vi "Modules - Machines.vi"(8 "error in":errorcluster) -> (0 "error out":errorcluster)   [LabVIEW 2019]
uses:
  Controls/Machine - Device Type.ctl
  Controls/Machine-state.ctl
  <vilib>/Utility/miscctls.llb/LVRowAndColumnTypeDef.ctl
  Controls/eFGV States.ctl
  Controls/UDP - Command.ctl
  Controls/FGV States.ctl
  Controls/Communication - Write Data.ctl
  Controls/Global - Data UDP.vi
  Controls/Global - IP Address.vi
  Controls/Global - Handle V1.vi
  Controls/Global - Device.vi
  Controls/Global - Comport.vi
  Controls/Global - Channel.vi
  Controls/Global - Unit.vi
  Controls/Global - Device Type.vi
  Controls/Global - Handle.vi
  Controls/Global - Rendezvous.vi
panel:
  out "Enum 2":T1
  out "Numeric":i32
  out "Status out":string[](array[string])
  out "Enum":T1
  out "Loop":i32
  out "Success":bool
  out "Which Button?":T2(ring)=enum."Center Button"
  in  "Settings":bool
  out "Device Type":string[](array[string])
  out "Device IP":string[](array[string])
  out "Label Ch2":string caption="Cell Pressure Transducer"
  out "Label Ch1":string caption="Cell Pressure Transducer"
  out "Channel 2":sgl format="%.2f"
  out "Channel 1":sgl caption="Kpa" format="%.3f"
  out "Label Ch4":string caption="Cell Pressure Transducer"
  out "Label Ch3":string caption="Cell Pressure Transducer"
  out "Channel 3":sgl format="%.2f"
  out "Channel 4":sgl caption="Kpa" format="%.2f"
  out "error out 2":errorcluster
  in  "Remove":bool
  in  "Add":bool
  in  "Table":i32(listbox)
  out "Main Tab":enum32{"Blank", "Edit"}(tab)
  in  "Machine Setting":bool
  out "Array":cluster{"Label":string, "Data":string}[](array[cluster])
  in  "Device Type":T3 items=["Unitron", "Flowtron", "Datalogger"]
  in  "Port":string
  in  "Device IP Address/SN":string
  in  "Device Name":string
  in  "Save Edit":bool
  in  "Refresh Button":bool
  in  "Reconnect":bool
  # "*Double-Click to Edit"
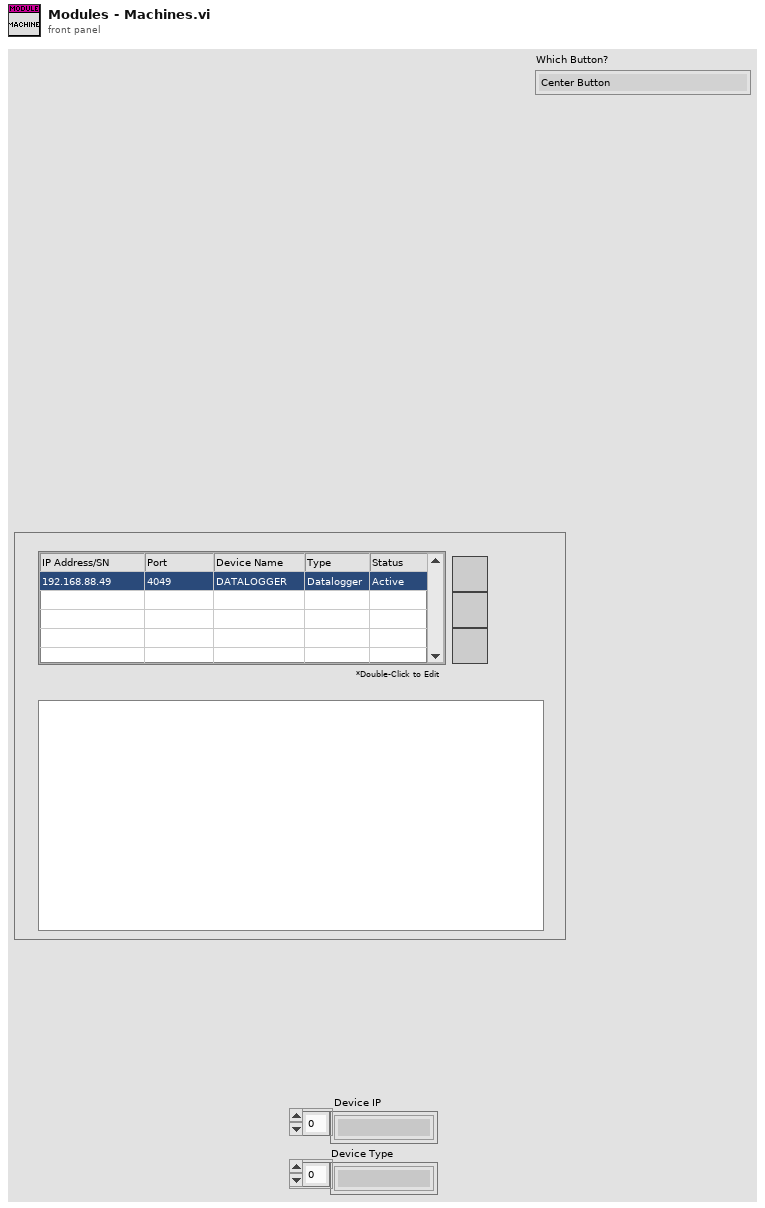
[diagram p1: front panel]
types:
  T1 = typedef "Machine-state.ctl" = enum16{"Init", "Read DB", "Read", "Idle", "Update", "Reset", "Close", "Exit"}
  T2 = enum16{"Left Button", "Center Button", "Right Button", "Window Close"}
  T3 = typedef "Machine - Device Type.ctl" = u16
  T4 = cluster{"Table":string[][], "no id":string, "doubleclick?":bool, "Timeout":i32, "Edit row":i32, "reset":i32}
  T5 = typedef "FGV States.ctl" = enum16{"Read", "Write"}
  T6 = enum32{"Invalid", "Standard", "Closed", "Hidden", "Minimized", "Maximized"}
  T7 = cluster{"Name":string[], "Unit":string[], "Decimal Point":u8[], "Ch Log":u8[], "H Alarm":u8[], "L Alarm":u8[], "H Limit":sgl[], "L Limit":sgl[], "Filter":u8[], "Gain":u8[], "Calib Type":u32[]}
  T8 = typedef "UDP - Command.ctl" = enum16{"Stop", "Jog Up", "Jog Down", "Ramp Up", "Ramp Down", "PID Target", "PID Ramp", "Disp Run", "Read Ch Data", "Zero Channel", "Zero Disp", "Read Sensor", "Write Sensor", "Read ADC", "Write ADC", "Read PID", "Write PID", "Read Test", "Write Test", "Read System", "Write System", "Read Datalog", "Read Datalog Sensor"}
  T9 = typedef "Communication - Write Data.ctl" = cluster{"Test":cluster{"Target Load":sgl, "Target Disp":sgl, "Rate":sgl, "Speed":sgl}, "Sensor":cluster{"Name":string[], "Unit":string[], "Decimal Point":u8[], "Ch Log":u8[], "H Alarm":u8[], "L Alarm":u8[], "H Limit":sgl[], "L Limit":sgl[], "Filter":u8[], "Gain":u8[], "Calib Type":u32[]}, "PID":cluster{"SP":sgl, "PV":sgl, "kP":sgl, "kI":sgl, "kD":sgl, "FF":sgl, "Err Band":sgl, "Max":i32, "Min":i32, "Ts":u32, "Out":i32, "Mode":u8}, "ADC":cluster{"Active Ch":u8[], "Filter Type":u8, "Post Filter":u8[], "Gain":u8[], "FS":u16, "IntOC":u8, "IntFC":u8, "SysOC":u8, "Cofficient":dbl[], "K":dbl[], "Max":i32}, "System":cluster{"Out Type":u8, "Inverse":u8, "Monitor":u8, "Reserve":u8, "ACC Time":u32, "Pulse Rev":u32, "Stroke":u32, "Auto Off":u32, "Gear Ratio":sgl, "Pitch":sgl, "Max Speed":u32, "Jog Speed":u32, "Disp Coff":sgl, "Max Load":u32}, "Index":enum16{"Ch1", "Ch2", "Ch3", "Ch4", "Ch5", "Ch6", "Ch7", "Ch8", "Ch9", "Ch10", "Ch11", "Ch12", "Ch13", "Ch14", "Ch15", "Ch16"}, "Datalog":enum16{"Ch1-Ch16", "Ch17-Ch32", "Ch32-Ch48", "Ch49-Ch64", "Empty"}}
  T10 = typedef "eFGV States.ctl" = enum16{"Init", "Read", "Write", "Exit"}
  T11 = typedef "Rendezvous RefNum" = refnum<k1>
  T12 = typedef "UDP - Event.ctl" = u16
  T13 = typedef "UDP - Status.ctl" = u16
  T14 = cluster{"Channels":cluster{"Ch1":sgl, "Ch2":sgl, "Ch3":sgl, "Ch4":sgl, "Ch5":sgl, "Ch6":sgl, "Ch7":sgl, "Ch8":sgl, "Ch9":sgl, "Ch10":sgl, "Ch11":sgl, "Ch12":sgl, "Ch13":sgl, "Ch14":sgl, "Ch15":sgl, "Ch16":sgl}, "Event":T12, "Status":T13, "IP":string}[]
  T15 = cluster{"Channels":cluster{"Ch1":sgl, "Ch2":sgl, "Ch3":sgl, "Ch4":sgl, "Ch5":sgl, "Ch6":sgl, "Ch7":sgl, "Ch8":sgl, "Ch9":sgl, "Ch10":sgl, "Ch11":sgl, "Ch12":sgl, "Ch13":sgl, "Ch14":sgl, "Ch15":sgl, "Ch16":sgl}, "Event":T12, "Status":T13, "IP":string}
  T16 = cluster{"Name":string[], "Unit":string[], "Decimal Point":u8[], "Ch Log":u8[], "H Alarm":u8[], "L Alarm":u8[], "H Limit":sgl[], "L Limit":sgl[], "Filter":u8[], "Gain":u8[], "Calib Type":u32[]}[]
  T17 = cluster{"Ch1":sgl, "Ch2":sgl, "Ch3":sgl, "Ch4":sgl, "Ch5":sgl, "Ch6":sgl, "Ch7":sgl, "Ch8":sgl, "Ch9":sgl, "Ch10":sgl, "Ch11":sgl, "Ch12":sgl, "Ch13":sgl, "Ch14":sgl, "Ch15":sgl, "Ch16":sgl}
  T18 = cluster{"Ch1 Unit":string, "Ch2 Unit":string, "Ch1 Decimal":u8, "Ch2 Decimal":u8, "Ch1 Cal Type":u8, "Ch2 Cal Type":u8}
  T19 = cluster{"IP Address":string, "port":string, "UDP ref":refnum<k16>}[]
  T20 = cluster{"IP Address":string, "port":string, "UDP ref":refnum<k16>}
  T21 = cluster{"Test":cluster{"Target Load":sgl, "Target Disp":sgl, "Rate":sgl, "Speed":sgl}, "Sensor":cluster{"Name":string[], "Unit":string[], "Decimal Point":u8[], "Ch Log":u8[], "H Alarm":u8[], "L Alarm":u8[], "H Limit":sgl[], "L Limit":sgl[], "Filter":u8[], "Gain":u8[], "Calib Type":u32[]}, "PID":cluster{"SP":sgl, "PV":sgl, "kP":sgl, "kI":sgl, "kD":sgl, "FF":sgl, "Err Band":sgl, "Max":i32, "Min":i32, "Ts":u32, "Out":i32, "Mode":u8}, "ADC":cluster{"Active Ch":u8[], "Filter Type":u8, "Post Filter":u8[], "Gain":u8[], "FS":u16, "IntOC":u8, "IntFC":u8, "SysOC":u8, "Cofficient":dbl[], "K":dbl[], "Max":i32}, "Status":T13, "Event":T12, "System":cluster{"Out Type":u8, "Inverse":u8, "Monitor":u8, "Reserve":u8, "ACC Time":u32, "Pulse Rev":u32, "Stroke":u32, "Auto Off":u32, "Gear Ratio":sgl, "Pitch":sgl, "Max Speed":u32, "Jog Speed":u32, "Disp Coff":sgl, "Max Load":u32}, "Channels":cluster{"Ch1":sgl, "Ch2":sgl, "Ch3":sgl, "Ch4":sgl, "Ch5":sgl, "Ch6":sgl, "Ch7":sgl, "Ch8":sgl, "Ch9":sgl, "Ch10":sgl, "Ch11":sgl, "Ch12":sgl, "Ch13":sgl, "Ch14":sgl, "Ch15":sgl, "Ch16":sgl}}
  T22 = typedef "LVRowAndColumnTypeDef.ctl" = cluster{"Row":i32, "Column":i32}
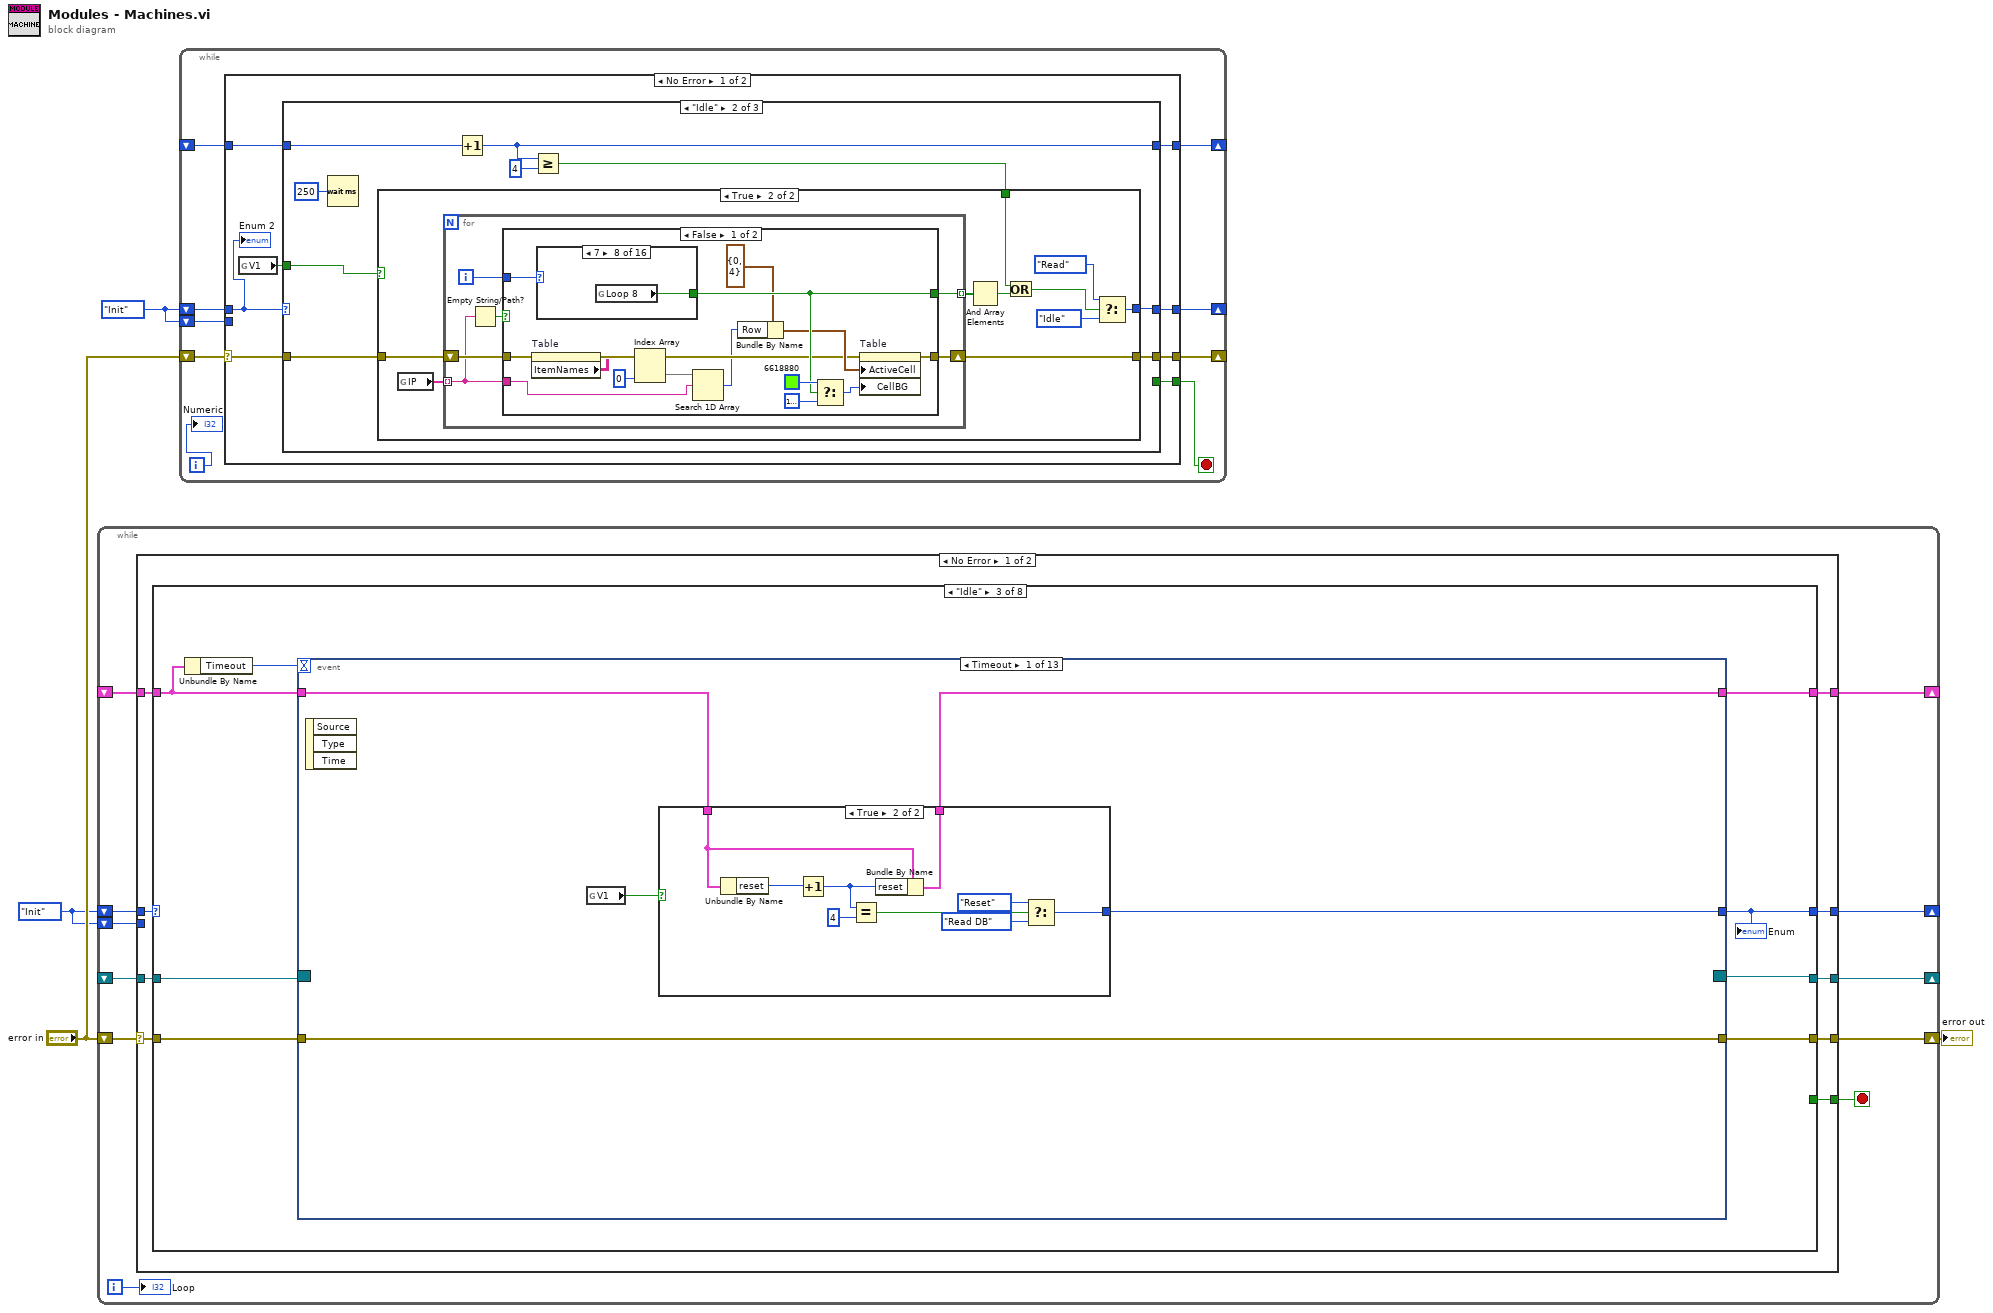
[diagram p0: block diagram]
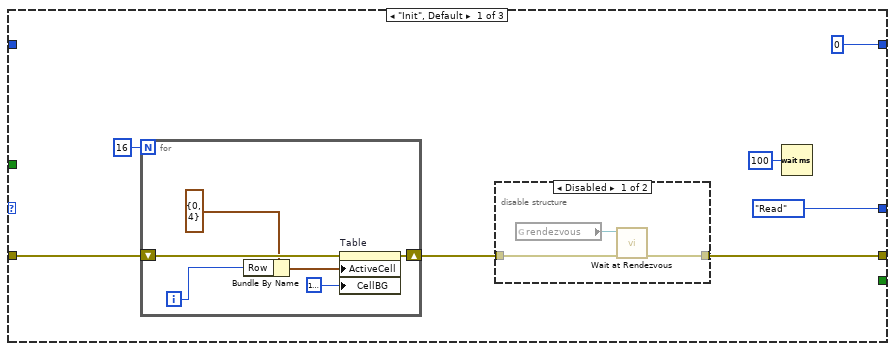
[diagram p2: hidden frame]
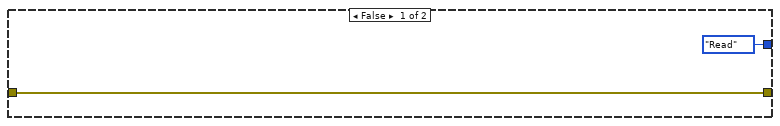
[diagram p4: hidden frame]
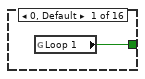
[diagram p5: hidden frame]
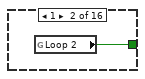
[diagram p6: hidden frame]
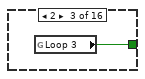
[diagram p7: hidden frame]
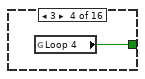
[diagram p8: hidden frame]
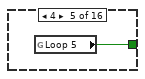
[diagram p9: hidden frame]
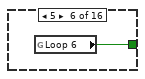
[diagram p10: hidden frame]
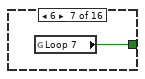
[diagram p11: hidden frame]
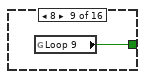
[diagram p12: hidden frame]
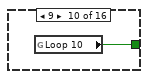
[diagram p13: hidden frame]
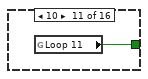
[diagram p14: hidden frame]
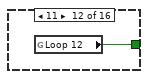
[diagram p15: hidden frame]
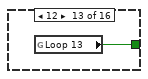
[diagram p16: hidden frame]
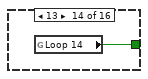
[diagram p17: hidden frame]
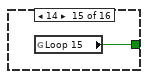
[diagram p18: hidden frame]
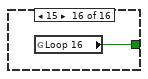
[diagram p19: hidden frame]
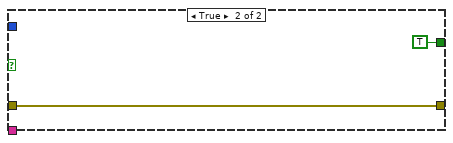
[diagram p20: hidden frame]
diagram:
  w1 = Machine-state."Init"
  w2 = Machine-state."Init"
  n1 = while {
    shift-right: [w14] -> w4
    shift-left: "error in" -> [w15]
    shift-right: [w12] -> _
    shift-left: w2 -> [w13]
    shift-right: [w10] -> _
    shift-left: _ -> [w9]
    shift-right: [w8] -> _
    shift-left: _ -> [w7]
    shift-left: w2 -> [w5]
    i -> [w6]
    stop <- w11 stop-if-true
    n2 = case shown="No Error" w15 {
      selector: w15 -> [w20 w611]
      tunnel: [w21 w612] -> w14
      tunnel: w13 -> [w24 _]
      tunnel: [w23 Machine-state."Idle"] -> w12
      tunnel: [w22 _] -> w11
      tunnel: [w19 w617] -> w10
      tunnel: w9 -> [w18 w617]
      tunnel: [w17 w614] -> w8
      tunnel: w7 -> [w16 w614]
      tunnel: w5 -> [_ w603]
      frame No Error {
        n3 = case shown="\"Idle\"" w24 {
          tunnel: [Machine-state."Read DB" Machine-state."Read" w127 Machine-state."Idle" Machine-state."Read DB" Machine-state."Idle" Machine-state."Idle" Machine-state."Exit"] -> w23
          tunnel: [_ _ _ _ _ _ FALSE TRUE] -> w22
          tunnel: [w39 w57 w129 w397 w477 w484 w588 w598] -> w21
          tunnel: w20 -> [w26 w75 w128 w401 w461 w483 w592 w597]
          tunnel: [T4 {"Table"=[], "no id"="", "doubleclick?"=FALSE, "Timeout"=1000, "Edit row"=-1, "reset"=0} w79 w126 w403 w472 w487 w591 w602] -> w19
          tunnel: w18 -> [_ w78 w123 w402 w472 w487 w591 w602]
          tunnel: [w36 w80 w124 w411 w482 w485 w589 w601] -> w17
          tunnel: w16 -> [_ w80 w125 w411 w482 w485 w589 w601]
          frame "Init", Default {
            w30 = eFGV_States."Read" ("Action")
            n4 = global read "Global - Data UDP.vi" "V1"() -> (w25:bool)
            n5 = property on="Reconnect" class="Bool"(error in=w26, "Visible"=w25) -> (error out=w27:errorcluster)  [unwired: 1 in, 1 out]
            n6 = Not(x=w25) -> (.not. x?=w28:bool)
            n7 = property on="Device Type" class="Ring (strict)"(error in=w27, "Visible"=w28) -> (error out=w29:errorcluster)  [unwired: 1 in, 1 out]
            n8 = disable-structure shown="Enabled" {
              disable-tunnel: w29 -> [w45 w47]
              disable-tunnel: [w44 w47] -> w33
              frame Disabled {
                n9 = global read "Global - Rendezvous.vi" "rendezvous"() -> (w46:T11)
                n10 = call <vilib>:"Wait at Rendezvous.vi"("error in (no error)"=w45, "rendezvous"=w46) -> ("error out"=w44:errorcluster)  [unwired: 3 in, 2 out]
              }
              frame Enabled {
              }
            }
            n11 = local write "Device Name"("" ("New machine name")) -> ()
            n12 = call "Main - Minimized (eFGV).vi"("Action"=w30, "error in"=w33) -> ("error out"=w32:errorcluster, "Minimized ref"=w31:refnum<user-event>)  [unwired: 7 in, 1 out]
            n13 = call "Communication - Trigger Read IP Address(FGV).vi"("Action"=w30, "error in"=w32) -> ("error out"=w35:errorcluster, "Trigger ref"=w34:refnum<user-event>)  [unwired: 7 in, 1 out]
            n14 = call "General - Exit eFGV.vi"("eFGV States"=w30, "error in (no error)"=w35) -> ("error out"=w40:errorcluster, "Exit"=w38:refnum<user-event>)  [unwired: 7 in, 1 out]
            n15 = register-events(error in=w40, w38, w34, w31) -> (reference out=w36:refnum<event-registration>, error out=w39:errorcluster)  [unwired: 1 in]
            "Main Tab" <- enum32{"Blank", "Edit"}."Blank" ("Main Tab")
          }
          frame "Read DB" {
            n16 = global read "Global - IP Address.vi" "IP"() -> (w48:string[])
            n17 = global read "Global - Data UDP.vi" "V1"() -> (w50:bool)
            n18 = call "Machine - Config File.vi"("Action"=enum16{"Write", "Read", "Read All", "Remove"}."Read All", "V1"=w50, "error in (no error)"=w75) -> ("error out"=w71:errorcluster, "Value Out"=w76:cluster{"IP/SN":string, "Key Value":string[]}[])  [unwired: 7 in]
            n19 = for {
              tunnel: [w113] -> w74 mode=indexing
              tunnel: w76 -> [w109] mode=indexing
              tunnel: [w102] -> w72 mode=indexing
              shift-right: [w107] -> w70
              shift-left: w71 -> [w108]
              tunnel: w48 -> [w94]
              n20 = Unbundle(w109) -> ("IP/SN"=w102:string, "Key Value"=w112:string[])
              n21 = Index Array(array=w112) -> (element #1=w101:string, element #2=w100:string, element #3=w93:string, element #4=w97:string)  [unwired: 4 in]
              n22 = Search 1D Array(1D array=w94, element=w102) -> (index of element=w96:i32)  [unwired: 1 in]
              n23 = Less Than 0?(x=w96) -> (x < 0?=w99:bool)
              n24 = Select(t="1" ("y"), s=w99, f="0") -> (s? t:f=w92:string)
              n25 = Select(t="Disable" ("y"), s=w99, f="Active" ("y")) -> (s? t:f=w98:string)
              n26 = Equal?(x=w92, y=w93) -> (x = y?=w91:bool)
              n27 = global read "Global - Data UDP.vi" "V1"() -> (w95:bool)
              n28 = Build Array(w92) -> (w103:string[])
              n29 = case shown="False" w91 {
                tunnel: w108 -> [w119 w121]
                tunnel: [w118 w121] -> w107
                tunnel: string[] ["Status"] ("Key Name") -> [w117 _]
                tunnel: w103 -> [w116 _]
                tunnel: w102 -> [w115 _]
                tunnel: w95 -> [w114 _]
                frame False {
                  n30 = call "Machine - Config File.vi"("Action"=enum16{"Write", "Read", "Read All", "Remove"}."Write", "V1"=w114, "error in (no error)"=w119, "Value"=w116, "Key Name"=w117, "IP/SN"=w115) -> ("error out"=w118:errorcluster)  [unwired: 4 in, 1 out]
                }
                frame True {
                }
              }
              n31 = Build Array(w101, w100, w97, w98) -> (w113:string[])
            }
            n32 = Empty Array?(array=w74) -> ()  [unwired: 1 out]
            n33 = case shown="False" FALSE {
              tunnel: [w85 w89] -> w68
              tunnel: w74 -> [w84 _]
              tunnel: [w83 w90] -> w73
              tunnel: w70 -> [w83 w90]
              tunnel: w72 -> [w82 _]
              frame False {
                n34 = Transpose 2D Array(2D array=w84) -> (transposed array=w86:string[][])
                n35 = Build Array (concatenate)(w82, w86) -> (w87:string[][])
                n36 = Transpose 2D Array(2D array=w87) -> (transposed array=w85:string[][])
              }
              frame True {
                n37 = global read "Global - IP Address.vi" "IP"() -> (w88:string[])
                n38 = Build Array(w88) -> (w89:string[][])
              }
            }
            n39 = property on="Table" class="MCListbox (strict)"(error in=w73, "ItemNames"=w68) -> (error out=w65:errorcluster)  [unwired: 1 in, 1 out]
            n40 = Bundle By Name(cluster=w78, "Table"=w68) -> (w79:T4)
            n41 = Index Array(array=w68, index (col) #1=3 ("disabled index (col)"), index (col) #2=0 ("disabled index (col)"), index (col) #3=2 ("disabled index (col)"), index (col) #4=4 ("index (col)")) -> (element #1=→"Device Type":string[], element #2=w53:string[], element #3=w62:string[], element #4=w63:string[])  [unwired: 4 in]
            "Device IP" <- w53
            n42 = call "Main - Machine Connectivity (FGV).vi"("Action"=FGV_States."Write", "error In"=w65, "Status"=w63, "Device Name"=w62) -> ("error out"=w58:errorcluster, "Status out"=→"Status out":string[])  [unwired: 5 in, 1 out]
            n43 = call "Communication - Heartbeat (FGV).vi"("Action"=FGV_States."Read", "error in (no error)"=w58) -> ("error out"=w59:errorcluster, "Previous Out"=w55:string[], "Timestamp Out"=w56:string[])  [unwired: 6 in, 1 out]
            n44 = call "Communication - Heartbeat (FGV).vi"("Action"=FGV_States."Write", "error in (no error)"=w59, "Previous"=w55, "Timestamp"=w56, "IP"=w53) -> ("error out"=w57:errorcluster)  [unwired: 3 in, 3 out]
          }
          frame "Idle" {
            n45 = Unbundle By Name(w123) -> ("Timeout"=w122:i32)
            n46 = event shown="[0] Timeout" {
              selector: w125 -> [_ _ _ _ _ _ _ _ _ _ _ _ _]
              dyn-events: [_ _ _ _ _ _ _ _ _ _ _ _ _] -> w124
              timeout: w122 -> [_ _ _ _ _ _ _ _ _ _ _ _ _]
              tunnel: [w134 w148 w149 w159 w169 w182 w211 w223 w241 w252 w326 w360 w388] -> w129
              tunnel: w128 -> [w134 w148 w150 w159 w168 w183 w211 w224 w242 w251 w340 w359 w388]
              tunnel: [w131 Machine-state."Close" Machine-state."Idle" Machine-state."Read DB" w170 Machine-state."Idle" Machine-state."Reset" w225 Machine-state."Read DB" Machine-state."Idle" Machine-state."Idle" Machine-state."Idle" Machine-state."Exit"] -> w127
              tunnel: w123 -> [w132 w147 w155 w158 w166 w184 w208 w222 w240 w265 w343 w362 w387]
              tunnel: [w133 w147 w155 w158 w166 w185 w209 w222 w240 w265 w343 w362 w387] -> w126
              event Timeout {
                n47 = event-data() -> ()  [unwired: 1 in, 3 out]
                n48 = global read "Global - Data UDP.vi" "V1"() -> (w130:bool)
                n49 = case shown="True" w130 {
                  tunnel: [w135 w143] -> w133
                  tunnel: w132 -> [w135 w142]
                  tunnel: [Machine-state."Read DB" w138] -> w131
                  frame False {
                  }
                  frame True {
                    n50 = Unbundle By Name(w142) -> ("reset"=w145:i32)
                    n51 = Increment(x=w145) -> (x+1=w141:i32)
                    n52 = Equal?(x=w141, y=4) -> (x = y?=w140:bool)
                    n53 = Bundle By Name(cluster=w142, "reset"=w141) -> (w143:T4)
                    n54 = Select(t=Machine-state."Reset", s=w140, f=Machine-state."Read DB") -> (s? t:f=w138:T1)
                  }
                }
              }
              event Panel Close {
                n55 = event-data() -> ()  [unwired: 1 in, 4 out]
              }
              event User Event {
                n56 = event-data() -> ()  [unwired: 1 in, 5 out]
                n57 = control-ref of="This VI"() -> (w153:refnum<vi>)
                n58 = property class="VI"(reference=w153, error in=w150, "FP.State"=T6."Minimized" ("Front Panel Window:State")) -> (error out=w151:errorcluster)  [unwired: 1 out]
                n59 = call <vilib>:"Clear Errors.vi"("error in (no error)"=w151) -> ("error out"=w149:errorcluster)  [unwired: 5 in, 1 out]
              }
              event User Event {
                n60 = event-data() -> ()  [unwired: 1 in, 5 out]
                n61 = Wait (ms)(milliseconds to wait=u32 3000) -> ()  [unwired: 1 out]
              }
              event "Save Edit": Value Change {
                n62 = event-data() -> ()  [unwired: 1 in, 1 out]
                n63 = Unbundle By Name(w166) -> ("Table"=w165:string[][])
                n64 = Index Array(array=w165, index (col)=1 ("disabled index (col)")) -> (element=w162:string[])  [unwired: 1 in]
                n65 = To Upper Case(1:"Device Name") -> (0:w161:string)
                n66 = Search 1D Array(1D array=w162, element=w161) -> (index of element=w160:i32)  [unwired: 1 in]
                n67 = case shown="-1" w160 {
                  tunnel: [w174 w181] -> w169
                  tunnel: w168 -> [w174 w181]
                  tunnel: [FALSE ("T button?") w177] -> w167
                  frame 0, Default {
                    n68 = One Button Dialog(message="This machine name already exist. Please give new name", button name ("OK")="Ok") -> ()  [unwired: 1 out]
                  }
                  frame -1 {
                    n69 = Two Button Dialog(message="Are you sure?", 1:"No" ("F button name (\"Cancel\")"), 2:"Yes" ("T button name (\"OK\")")) -> (T button?=w177:bool)
                  }
                }
                n70 = Select(t=Machine-state."Update", s=w167, f=Machine-state."Idle") -> (s? t:f=w170:T1)
              }
              event "Table": Mouse Down {
                n71 = event-data() -> ("Mods.Double Click"=w187:bool)  [unwired: 1 in]
                n72 = case shown="True" w187 {
                  tunnel: w184 -> [w189 w192]
                  tunnel: [w189 w193] -> w185
                  tunnel: w183 -> [w188 w200]
                  tunnel: [w188 w200] -> w182
                  frame False {
                  }
                  frame True {
                    n73 = Unbundle By Name(w192) -> ("Table"=w203:string[][])
                    n74 = Index Array(array=w203, index (row) #1="Table", index (col) #1=0 ("disabled index (col)"), index (row) #2="Table", index (col) #2=1 ("disabled index (col)"), index (row) #3="Table", index (col) #3=2 ("disabled index (col)"), index (row) #4="Table", index (col) #4=3 ("disabled index (col)")) -> (element #1=w194:string, element #2=w190:string, element #3=w199:string, element #4=w196:string)
                    n75 = case shown="\"Datalogger\"" w196 {
                      tunnel: [w205 w206 w207] -> w195
                      frame "Unitron", Default {
                        w205 = T3 0 items=["Unitron", "Flowtron", "Datalogger"] ("Device Type")
                      }
                      frame "Flowtron" {
                        w206 = T3 1 items=["Unitron", "Flowtron", "Datalogger"] ("Device Type")
                      }
                      frame "Datalogger" {
                        w207 = T3 2 items=["Unitron", "Flowtron", "Datalogger"] ("Device Type")
                      }
                    }
                    n76 = local write "Device IP Address/SN"(w194) -> ()
                    n77 = local write "Device Name"(w199) -> ()
                    n78 = local write "Port"(w190) -> ()
                    n79 = Bundle By Name(cluster=w192, "Edit row"="Table") -> (w193:T4)
                    n80 = local write "Device Type"(w195) -> ()
                    n81 = local write "Main Tab"(enum32{"Blank", "Edit"}."Edit" ("Main Tab")) -> ()
                  }
                }
              }
              event "Refresh Button": Value Change {
                n82 = event-data() -> ()  [unwired: 1 in, 6 out]
                n83 = Bundle By Name(cluster=w208, "Timeout"=1000) -> (w209:T4)
              }
              event "Add": Value Change {
                n84 = event-data() -> ()  [unwired: 1 in, 6 out]
                n85 = Unbundle By Name(w222) -> ("Table"=w217:string[][])
                n86 = Array Size(array=w217) -> (size(s)=w221:i32[])
                n87 = Index Array(array=w221) -> (element=w220:i32)  [unwired: 1 in]
                n88 = Index Array(array=w217, index (col) #1=1 ("disabled index (col)"), index (col) #2=0 ("index (col)")) -> (element #1=w213:string[], element #2=w214:string[])  [unwired: 2 in]
                n89 = Greater Or Equal?(x=w220, y=16) -> (x >= y?=w218:bool)
                n90 = case shown="False" w218 {
                  tunnel: [Machine-state."Read DB" Machine-state."Idle"] -> w225
                  tunnel: w224 -> [w229 w232]
                  tunnel: [w228 w232] -> w223
                  tunnel: w214 -> [w227 _]
                  tunnel: w213 -> [w226 _]
                  frame False {
                    n91 = call "Machine - Add Device (SubVI).vi"("error in"=w229, "IP Address/SN"=w227, "Port"=w226) -> ("error out"=w228:errorcluster)  [unwired: 8 in]
                  }
                  frame True {
                    n92 = One Button Dialog(message="Maximum devices already reached") -> ()  [unwired: 1 in, 1 out]
                  }
                }
              }
              event "Remove": Value Change {
                n93 = event-data() -> ()  [unwired: 1 in, 6 out]
                n94 = local read "Table"() -> (w237:i32)
                n95 = Unbundle By Name(w240) -> ("Table"=w239:string[][])
                n96 = Two Button Dialog(message="Are your sure?") -> (T button?=w235:bool)  [unwired: 2 in]
                n97 = Index Array(array=w239, index (row)=w237, index (col)=0 ("disabled index (col)")) -> (element=w236:string)
                n98 = case shown="True" w235 {
                  tunnel: w242 -> [w244 w248]
                  tunnel: [w244 w247] -> w241
                  tunnel: w236 -> [_ w246]
                  frame False {
                  }
                  frame True {
                    n99 = global read "Global - Data UDP.vi" "V1"() -> (w245:bool)
                    n100 = call "Machine - Config File.vi"("Action"=enum16{"Write", "Read", "Read All", "Remove"}."Remove", "V1"=w245, "error in (no error)"=w248, "IP/SN"=w246) -> ("error out"=w247:errorcluster)  [unwired: 6 in, 1 out]
                  }
                }
              }
              event "Settings": Value Change {
                n101 = event-data() -> ()  [unwired: 1 in, 6 out]
                n102 = global read "Global - Data UDP.vi" "V1"() -> (w262:bool)
                n103 = Select(t="USB" ("message"), s=w262, f="LAN" ("message")) -> (s? t:f=w259:string)
                n104 = Format Into String(format string="Currently the system run \"%s\" communication protocol.\nSelect the Communication protocol you want to use." ("message"), initial string="", w259) -> (resulting string=w257:string)  [unwired: 1 in, 1 out]
                n105 = call <vilib>:"Three Button Dialog.vi"("Justify Message (Left)"=enum16{"Left", "Center", "Right"}."Center", "Window Title (\"\")"="Communication Protocol" ("Window Title (\"\")"), "Center Button Text (\"No\")"="LAN" ("Center Button Text (\"No\")"), "Left Button Text (\"Yes\")"="USB" ("Left Button Text (\"Yes\")"), "message"=w257) -> ("Which Button?"=w250:T2)  [unwired: 6 in]
                "Which Button?" <- w250
                n106 = case shown="\"Right Button\"" w250 {
                  tunnel: [w272 w280 w283 w304] -> w252
                  tunnel: w251 -> [w271 w279 w283 w304]
                  frame "Center Button", Default {
                    n107 = call "Machine - Config File.vi"("Setting"=TRUE, "Action"=enum16{"Write", "Read", "Read All", "Remove"}."Write", "error in (no error)"=w271, "Value"=string[] ["V2"], "Key Name"=string[] ["Controller"], "IP/SN"="Setting") -> ("error out"=w272:errorcluster)  [unwired: 4 in, 1 out]
                    n108 = One Button Dialog(message="Restart the sytem to enable the changes.") -> ()  [unwired: 1 in, 1 out]
                  }
                  frame "Left Button" {
                    n109 = call "Machine - Config File.vi"("Setting"=TRUE, "Action"=enum16{"Write", "Read", "Read All", "Remove"}."Write", "error in (no error)"=w279, "Value"=string[] ["V1"], "Key Name"=string[] ["Controller"], "IP/SN"="Setting") -> ("error out"=w280:errorcluster)  [unwired: 4 in, 1 out]
                    n110 = One Button Dialog(message="Restart the sytem to enable the changes.") -> ()  [unwired: 1 in, 1 out]
                  }
                  frame "Right Button" {
                    n111 = global read "Global - IP Address.vi" "IP"() -> (w282:string[])
                    n112 = for {
                      tunnel: w282 -> [w284] mode=indexing
                      i -> [w285]
                      n113 = case shown="Default" w284 {
                        tunnel: w285 -> [w286 _]
                        frame Default {
                          n114 = case shown="12" w286 {
                            frame 0, Default {
                              n115 = global write "Global - Data UDP.vi" "Loop 1"(TRUE ("Loop 1")) -> ()
                            }
                            frame 1 {
                              n116 = global write "Global - Data UDP.vi" "Loop 2"(TRUE ("Loop 2")) -> ()
                            }
                            frame 2 {
                              n117 = global write "Global - Data UDP.vi" "Loop 3"(TRUE ("Loop 3")) -> ()
                            }
                            frame 3 {
                              n118 = global write "Global - Data UDP.vi" "Loop 4"(TRUE ("Loop 4")) -> ()
                            }
                            frame 4 {
                              n119 = global write "Global - Data UDP.vi" "Loop 5"(TRUE ("Loop 5")) -> ()
                            }
                            frame 5 {
                              n120 = global write "Global - Data UDP.vi" "Loop 6"(TRUE ("Loop 6")) -> ()
                            }
                            frame 6 {
                              n121 = global write "Global - Data UDP.vi" "Loop 7"(TRUE ("Loop 7")) -> ()
                            }
                            frame 7 {
                              n122 = global write "Global - Data UDP.vi" "Loop 8"(TRUE ("Loop 8")) -> ()
                            }
                            frame 8 {
                              n123 = global write "Global - Data UDP.vi" "Loop 9"(TRUE ("Loop 9")) -> ()
                            }
                            frame 9 {
                              n124 = global write "Global - Data UDP.vi" "Loop 10"(TRUE ("Loop 10")) -> ()
                            }
                            frame 10 {
                              n125 = global write "Global - Data UDP.vi" "Loop 11"(TRUE ("Loop 11")) -> ()
                            }
                            frame 11 {
                              n126 = global write "Global - Data UDP.vi" "Loop 12"(TRUE ("Loop 12")) -> ()
                            }
                            frame 12 {
                              n127 = global write "Global - Data UDP.vi" "Loop 13"(TRUE ("Loop 13")) -> ()
                            }
                            frame 13 {
                              n128 = global write "Global - Data UDP.vi" "Loop 14"(TRUE ("Loop 14")) -> ()
                            }
                            frame 14 {
                              n129 = global write "Global - Data UDP.vi" "Loop 15"(TRUE ("Loop 15")) -> ()
                            }
                            frame 15 {
                              n130 = global write "Global - Data UDP.vi" "Loop 16"(TRUE ("Loop 16")) -> ()
                            }
                          }
                        }
                        frame "" {
                        }
                      }
                    }
                  }
                  frame "Window Close" {
                    n131 = global read "Global - IP Address.vi" "IP"() -> (w303:string[])
                    n132 = for {
                      tunnel: w303 -> [w305] mode=indexing
                      i -> [w306]
                      n133 = case shown="Default" w305 {
                        tunnel: w306 -> [w307 _]
                        frame Default {
                          n134 = case shown="8" w307 {
                            frame 0, Default {
                              n135 = global write "Global - Data UDP.vi" "Loop 1"(TRUE ("Loop 1")) -> ()
                            }
                            frame 1 {
                              n136 = global write "Global - Data UDP.vi" "Loop 2"(TRUE ("Loop 2")) -> ()
                            }
                            frame 2 {
                              n137 = global write "Global - Data UDP.vi" "Loop 3"(TRUE ("Loop 3")) -> ()
                            }
                            frame 3 {
                              n138 = global write "Global - Data UDP.vi" "Loop 4"(TRUE ("Loop 4")) -> ()
                            }
                            frame 4 {
                              n139 = global write "Global - Data UDP.vi" "Loop 5"(TRUE ("Loop 5")) -> ()
                            }
                            frame 5 {
                              n140 = global write "Global - Data UDP.vi" "Loop 6"(TRUE ("Loop 6")) -> ()
                            }
                            frame 6 {
                              n141 = global write "Global - Data UDP.vi" "Loop 7"(TRUE ("Loop 7")) -> ()
                            }
                            frame 7 {
                              n142 = global write "Global - Data UDP.vi" "Loop 8"(TRUE ("Loop 8")) -> ()
                            }
                            frame 8 {
                              n143 = global write "Global - Data UDP.vi" "Loop 9"(TRUE ("Loop 9")) -> ()
                            }
                            frame 9 {
                              n144 = global write "Global - Data UDP.vi" "Loop 10"(TRUE ("Loop 10")) -> ()
                            }
                            frame 10 {
                              n145 = global write "Global - Data UDP.vi" "Loop 11"(TRUE ("Loop 11")) -> ()
                            }
                            frame 11 {
                              n146 = global write "Global - Data UDP.vi" "Loop 12"(TRUE ("Loop 12")) -> ()
                            }
                            frame 12 {
                              n147 = global write "Global - Data UDP.vi" "Loop 13"(TRUE ("Loop 13")) -> ()
                            }
                            frame 13 {
                              n148 = global write "Global - Data UDP.vi" "Loop 14"(TRUE ("Loop 14")) -> ()
                            }
                            frame 14 {
                              n149 = global write "Global - Data UDP.vi" "Loop 15"(TRUE ("Loop 15")) -> ()
                            }
                            frame 15 {
                              n150 = global write "Global - Data UDP.vi" "Loop 16"(TRUE ("Loop 16")) -> ()
                            }
                          }
                        }
                        frame "" {
                        }
                      }
                    }
                  }
                }
              }
              event "Reconnect": Value Change {
                n151 = event-data() -> ()  [unwired: 1 in, 1 out]
                n152 = local read "Device IP Address/SN"() -> (w342:string)
                n153 = global read "Global - Handle V1.vi" "Handle"() -> (w330:refnum<visa-resource-name>[])
                n154 = global read "Global - IP Address.vi" "IP"() -> (w341:string[])
                n155 = Search 1D Array(1D array=w341, element=w342) -> (index of element=w325:i32)  [unwired: 1 in]
                n156 = Index Array(array=w341, index=w325) -> (element=w337:string)
                n157 = Index Array(array=w330, index=w325) -> (element=w339:refnum<visa-resource-name>)
                n158 = VISA Close(VISA resource name=w339, error in (no error)=w340) -> (error out=w331:errorcluster)
                n159 = flat-sequence {
                  tunnel: [w357] -> w332
                  tunnel: w331 -> [w357]
                  frame #0 {
                    n160 = Wait (ms)(milliseconds to wait=u32 250) -> ()  [unwired: 1 out]
                  }
                }
                n161 = call "FTDI - Read Registry.vi"("error in (no error)"=w332) -> ("error out"=w334:errorcluster, "Serial Number"=w338:string[], "ComPort"=w336:string[])  [unwired: 8 in]
                n162 = Search 1D Array(1D array=w338, element=w337) -> (index of element=w335:i32)  [unwired: 1 in]
                n163 = Index Array(array=w336, index=w335) -> (element=w333:string)
                n164 = call "VISA - Open Connection.vi"("error in"=w334, "VISA resource name"=w333) -> ("error out"=w327:errorcluster, "VISA Ref"=w329:refnum<visa-resource-name>)  [unwired: 8 in]
                n165 = Replace Array Subset(array=w330, new element=w329, index=w325) -> (w328:refnum<visa-resource-name>[])
                n166 = global write "Global - Handle V1.vi" "Handle"(w328) -> ()
                n167 = case shown="No Error" w327 {
                  selector: w327 -> [w344 w356]
                  tunnel: [w344 w355] -> w326
                  tunnel: w325 -> [_ w350]
                  frame No Error {
                  }
                  frame Error {
                    w345 = "" ("new element/subarray")
                    n168 = global read "Global - Handle V1.vi" "Handle"() -> (w353:refnum<visa-resource-name>[])
                    n169 = global read "Global - Device.vi" "Device"() -> (w351:string[])
                    n170 = global read "Global - Comport.vi" "Port"() -> (w352:string[])
                    n171 = global read "Global - IP Address.vi" "IP"() -> (w354:string[])
                    n172 = Replace Array Subset(array=w354, new element=w345, index=w350) -> (w349:string[])
                    n173 = Replace Array Subset(array=w353, new element=w345, index=w350) -> (w348:refnum<visa-resource-name>[])
                    n174 = Replace Array Subset(array=w352, new element=w345, index=w350) -> (w347:string[])
                    n175 = Replace Array Subset(array=w351, new element=w345, index=w350) -> (w346:string[])
                    n176 = global write "Global - IP Address.vi" "IP"(w349) -> ()
                    n177 = global write "Global - Handle V1.vi" "Handle"(w348) -> ()
                    n178 = global write "Global - Comport.vi" "Port"(w347) -> ()
                    n179 = global write "Global - Device.vi" "Device"(w346) -> ()
                    n180 = call <vilib>:"Clear Errors.vi"("error in (no error)"=w356) -> ("error out"=w355:errorcluster)  [unwired: 5 in, 1 out]
                  }
                }
              }
              event "Machine Setting": Value Change {
                n181 = event-data() -> ()  [unwired: 1 in, 6 out]
                n182 = disable-structure shown="Disabled" {
                  disable-tunnel: [w368 w385] -> w360
                  disable-tunnel: w359 -> [w365 w385]
                  frame Disabled {
                    # "#todo: create popup to setup PID like controller software"
                    n183 = call "Main - Root Path (FGV).vi"("Action"=FGV_States."Read", "error in"=w365) -> ("error out"=w366:errorcluster, "Path out"=w364:path)  [unwired: 8 in]
                    n184 = local read "Device IP Address/SN"() -> (w363:string)
                    n185 = Build Path(base path=w364, name or relative path="SubVIs") -> (appended path=w383:path)
                    n186 = Build Path(base path=w383, name or relative path="Report - Generate Report.vi") -> (appended path=w384:path)
                    n187 = Open VI Reference(vi path=w384, error in (no error)=w366) -> (vi reference=w370:refnum<vi>, error out=w373:errorcluster)  [unwired: 4 in]
                    n188 = invoke class="VI" method="Ctrl Val.Set"(reference=w370, error in=w373, "Control Name"="IP Address", "Value"=w363) -> (reference out=w371:refnum<vi>, error out=w372:errorcluster)  [unwired: 1 in, 3 out]
                    n189 = invoke class="VI" method="Run VI"(reference=w371, error in=w372, "Wait until done"=FALSE ("Wait Until Done"), "Auto Dispose Ref"=FALSE ("Auto Dispose Reference")) -> (reference out=w382:refnum<vi>, error out=w381:errorcluster)  [unwired: 1 in, 3 out]
                    n190 = invoke class="VI" method="FP.Open"(reference=w382, error in=w381, "Activate"=TRUE ("Activate?"), "State"=T6."Standard") -> (error out=w369:errorcluster)  [unwired: 1 in, 4 out]
                    n191 = call <vilib>:"Simple Error Handler.vi"("error in (no error)"=w369) -> ("error out"=w368:errorcluster)  [unwired: 4 in, 4 out]
                  }
                  frame Enabled {
                  }
                }
              }
              event User Event {
                n192 = event-data() -> ()  [unwired: 1 in, 5 out]
              }
            }
            "Enum" <- w127
          }
          frame "Read" {
            n193 = local read "Device IP Address/SN"() -> (w409:string)
            n194 = global read "Global - IP Address.vi" "IP"() -> (w389:string[])
            n195 = global read "Global - Channel.vi" "Data"() -> (w390:T14)
            n196 = Search 1D Array(1D array=w389, element=w409) -> (index of element=w406:i32)  [unwired: 1 in]
            n197 = Index Array(array=w390, index=w406) -> (element=w408:T15)
            n198 = global read "Global - Unit.vi" "Unit"() -> (w405:T16)
            n199 = Unbundle By Name(w408) -> ("Channels.Ch1"=→"Channel 1":sgl, "Channels.Ch2"=→"Channel 2":sgl, "Channels.Ch3"=→"Channel 4":sgl, "Channels.Ch4"=→"Channel 3":sgl, "Channels"=w396:T17)
            n200 = Index Array(array=w405, index=w406) -> (element=w407:T7)
            n201 = Unbundle By Name(w407) -> ("Name"=w399:string[], "Unit"=w400:string[], "Decimal Point"=w398:u8[])
            n202 = Cluster To Array(cluster=w396) -> (array=w395:sgl[])
            n203 = disable-structure shown="Enabled" {
              disable-tunnel: w401 -> [w416 w448]
              disable-tunnel: w400 -> [w415 w446]
              disable-tunnel: w399 -> [w414 w447]
              disable-tunnel: w398 -> [w413 w444]
              disable-tunnel: [w412 w449] -> w397
              disable-tunnel: w395 -> [_ w445]
              frame Disabled {
                n204 = for {
                  shift-right: [w419] -> w412
                  shift-left: w416 -> [w422]
                  tunnel: w415 -> [w420] mode=indexing
                  tunnel: w414 -> [w421] mode=indexing
                  tunnel: w413 -> [w417] mode=indexing
                  i -> [w424]
                  n205 = Format Into String(format string="%s: (%s)", initial string="", error in=w422, w421, w420) -> (resulting string=w423:string, error out=w418:errorcluster)
                  n206 = case shown="0, Default" w424 {
                    tunnel: w423 -> [w430 w434 w438 w442]
                    tunnel: [w428 w432 w435 w440] -> w419
                    tunnel: w418 -> [w429 w433 w437 w441]
                    tunnel: w417 -> [w427 w431 w436 w439]
                    frame 0, Default {
                      n207 = property on="Channel 1" class="DigNum (strict)"(error in=w429, "Precision"=w427) -> (error out=w428:errorcluster)  [unwired: 1 in, 1 out]
                      "Label Ch1" <- w430
                    }
                    frame 1 {
                      n208 = property on="Channel 2" class="DigNum (strict)"(error in=w433, "Precision"=w431) -> (error out=w432:errorcluster)  [unwired: 1 in, 1 out]
                      "Label Ch2" <- w434
                    }
                    frame 2 {
                      n209 = property on="Channel 3" class="DigNum (strict)"(error in=w437, "Precision"=w436) -> (error out=w435:errorcluster)  [unwired: 1 in, 1 out]
                      "Label Ch3" <- w438
                    }
                    frame 3 {
                      n210 = property on="Channel 4" class="DigNum (strict)"(error in=w441, "Precision"=w439) -> (error out=w440:errorcluster)  [unwired: 1 in, 1 out]
                      "Label Ch4" <- w442
                    }
                  }
                }
              }
              frame Enabled {
                n211 = for {
                  shift-right: [w457] -> w449
                  shift-left: w448 -> [w458]
                  tunnel: w447 -> [w456] mode=indexing
                  tunnel: w446 -> [w455] mode=indexing
                  tunnel: w445 -> [w454] mode=indexing
                  tunnel: w444 -> [w453] mode=indexing
                  tunnel: [w451] -> w443 mode=indexing
                  n212 = Format Into String(format string="%s: (%s)", initial string="", error in=w458, w456, w455) -> (resulting string=w452:string, error out=w457:errorcluster)
                  n213 = Number To Fractional String(number=w454, precision (6)=w453) -> (F-format string=w450:string)  [unwired: 2 in]
                  n214 = Bundle(w452, w450) -> (w451:cluster{string, string})  [unwired: 1 in]
                }
                "Array" <- w443
              }
            }
            n215 = Bundle By Name(cluster=w402, "Timeout"=1000) -> (w403:T4)
          }
          frame "Update" {
            # "Type (0 - Unitron, 1 - Flowtron)"
            # "Type (0 - Unitron, 1 - Flowtron)"
            n216 = Unbundle By Name(w472) -> ("Table"=w471:string[][], "Edit row"=w470:i32)
            n217 = Index Array(array=w471, index (row)=w470, index (col)=0 ("disabled index (col)")) -> ()  [unwired: 1 out]
            n218 = global read "Global - Data UDP.vi" "V1"() -> (w468:bool)
            n219 = local read "Device Name"() -> (w475:string)
            n220 = property on="Device Type" class="Ring (strict)"(error in=w461) -> (error out=w474:errorcluster, "RingText.Text"=w467:string)  [unwired: 1 in, 1 out]
            n221 = To Upper Case(1:w475) -> (0:w464:string)
            n222 = Select(t="N/A", s=w468, f=w467) -> (s? t:f=w463:string)
            n223 = Build Array("Port", w464, "1" ("element"), w463) -> (w481:string[])
            n224 = call "Machine - Config File.vi"("Action"=enum16{"Write", "Read", "Read All", "Remove"}."Write", "V1"=w468, "error in (no error)"=w474, "Value"=w481, "Key Name"=string[] ["Port", "Device Name", "Status", "Type"], "IP/SN"="Device IP Address/SN") -> ("error out"=w477:errorcluster)  [unwired: 4 in, 1 out]
            n225 = local write "Main Tab"(enum32{"Blank", "Edit"}."Blank" ("Main Tab")) -> ()
          }
          frame "Reset" {
            n226 = disable-structure shown="Enabled" {
              disable-tunnel: [w489 w562] -> w484
              disable-tunnel: w483 -> [w488 w563]
              frame Disabled {
                n227 = global read "Global - Comport.vi" "Port"() -> (w490:string[])
                n228 = local read "Port"() -> (w492:string)
                n229 = Empty String/Path?(string/path=w492) -> (empty?=w491:bool)
                n230 = Search 1D Array(1D array=w490, element=w492) -> (index of element=w493:i32)  [unwired: 1 in]
                n231 = case shown="False" w491 {
                  tunnel: w493 -> [w498 _]
                  tunnel: [w496 w528] -> w489
                  tunnel: w488 -> [w494 w527]
                  tunnel: w490 -> [_ w526]
                  frame False {
                    n232 = global read "Global - Data UDP.vi" "V1"() -> (w495:bool)
                    n233 = case shown="False" w495 {
                      tunnel: w494 -> [w515 w525]
                      tunnel: [w514 w524] -> w496
                      tunnel: w498 -> [w517 w523]
                      tunnel: [w502 w518] -> w497
                      frame True {
                        n234 = global read "Global - Handle V1.vi" "Handle"() -> (w516:refnum<visa-resource-name>[])
                        n235 = Index Array(array=w516, index=w517) -> (element=w512:refnum<visa-resource-name>)
                        n236 = call "VISA - Write CMD.vi"("error in"=w515, "Action"=UDP_-_Command."Read Sensor", "VISA ref"=w512) -> ("error out"=w514:errorcluster, "Data Unit"=w503:T18, "Success"=→"Success":bool)  [unwired: 3 in, 3 out]
                        n237 = Unbundle By Name(w503) -> ("Ch1 Unit"=w510:string, "Ch2 Unit"=w509:string, "Ch1 Decimal"=w508:u8, "Ch2 Decimal"=w507:u8)
                        n238 = Build Array(w510, w509) -> (w506:string[])
                        n239 = Build Array(w508, w507) -> (w505:u8[])
                        n240 = Bundle By Name(cluster=T7 {"Name"=[], "Unit"=[], "Decimal Point"=[], "Ch Log"=[], "H Alarm"=[], "L Alarm"=[], "H Limit"=[], "L Limit"=[], "Filter"=[], "Gain"=[], "Calib Type"=[]} ("Sensor"), "Name"=string[] ["Load", "Displacement"], "Unit"=w506, "Decimal Point"=w505) -> (w502:T7)
                      }
                      frame False {
                        n241 = global read "Global - Handle.vi" "Handle"() -> (w522:T19)
                        n242 = Index Array(array=w522, index=w523) -> (element=w521:T20)
                        n243 = call "UDP - Write CMD.vi"("CMD"=UDP_-_Command."Read Sensor", "error in"=w525, "UDP Info"=w521) -> ("error out"=w524:errorcluster, "Data Out"=w519:T21)  [unwired: 2 in, 5 out]
                        n244 = Unbundle By Name(w519) -> ("Sensor"=w518:T7)
                      }
                    }
                    "error out 2" <- w496
                    n245 = global read "Global - Unit.vi" "Unit"() -> (w500:T16)
                    n246 = Replace Array Subset(array=w500, new element=w497, index=w498) -> (w499:T16)
                    n247 = global write "Global - Unit.vi" "Unit"(w499) -> ()
                  }
                  frame True {
                    n248 = for {
                      shift-right: [w532] -> w528
                      shift-left: w527 -> [w530]
                      tunnel: w526 -> [_] mode=indexing
                      i -> [w529]
                      n249 = global read "Global - Data UDP.vi" "V1"() -> (w531:bool)
                      n250 = case shown="True" w531 {
                        tunnel: w530 -> [w550 w560]
                        tunnel: [w549 w559] -> w532
                        tunnel: w529 -> [w552 w558]
                        tunnel: [w537 w553] -> w533
                        frame True {
                          n251 = global read "Global - Handle V1.vi" "Handle"() -> (w551:refnum<visa-resource-name>[])
                          n252 = Index Array(array=w551, index=w552) -> (element=w547:refnum<visa-resource-name>)
                          n253 = call "VISA - Write CMD.vi"("error in"=w550, "Action"=UDP_-_Command."Read Sensor", "VISA ref"=w547) -> ("error out"=w549:errorcluster, "Data Unit"=w538:T18, "Success"=w536:bool)  [unwired: 3 in, 3 out]
                          n254 = Unbundle By Name(w538) -> ("Ch1 Unit"=w545:string, "Ch2 Unit"=w544:string, "Ch1 Decimal"=w543:u8, "Ch2 Decimal"=w542:u8)
                          n255 = Build Array(w545, w544) -> (w541:string[])
                          n256 = Build Array(w543, w542) -> (w540:u8[])
                          n257 = local write "Success"(w536) -> ()
                          n258 = Bundle By Name(cluster=T7 {"Name"=[], "Unit"=[], "Decimal Point"=[], "Ch Log"=[], "H Alarm"=[], "L Alarm"=[], "H Limit"=[], "L Limit"=[], "Filter"=[], "Gain"=[], "Calib Type"=[]} ("Sensor"), "Name"=string[] ["Load", "Displacement"], "Unit"=w541, "Decimal Point"=w540) -> (w537:T7)
                        }
                        frame False {
                          n259 = global read "Global - Handle.vi" "Handle"() -> (w557:T19)
                          n260 = Index Array(array=w557, index=w558) -> (element=w556:T20)
                          n261 = call "UDP - Write CMD.vi"("CMD"=UDP_-_Command."Read Sensor", "error in"=w560, "UDP Info"=w556) -> ("error out"=w559:errorcluster, "Data Out"=w554:T21)  [unwired: 2 in, 5 out]
                          n262 = Unbundle By Name(w554) -> ("Sensor"=w553:T7)
                        }
                      }
                      n263 = global read "Global - Unit.vi" "Unit"() -> (w535:T16)
                      n264 = Replace Array Subset(array=w535, new element=w533, index=w529) -> (w534:T16)
                      n265 = global write "Global - Unit.vi" "Unit"(w534) -> ()
                    }
                  }
                }
              }
              frame Enabled {
                n266 = global read "Global - Device Type.vi" "Datalog"() -> (w561:bool[])
                n267 = global read "Global - Handle.vi" "Handle"() -> (w564:T19)
                n268 = for {
                  shift-right: [w567] -> w562
                  shift-left: w563 -> [w568]
                  tunnel: w564 -> [w566] mode=indexing
                  tunnel: w561 -> [w565] mode=indexing
                  n269 = case shown="False" w565 {
                    tunnel: w568 -> [w574 w578]
                    tunnel: [w573 w577] -> w567
                    tunnel: w566 -> [w571 w576]
                    frame False {
                      n270 = call "UDP - Write CMD.vi"("V2"=TRUE, "CMD"=UDP_-_Command."Read Sensor", "error in"=w574, "UDP Info"=w571) -> ("error out"=w573:errorcluster)  [unwired: 1 in, 6 out]
                      n271 = Wait (ms)(milliseconds to wait=u32 10) -> ()  [unwired: 1 out]
                    }
                    frame True {
                      n272 = for {
                        N: 16 -> [_]
                        tunnel: w576 -> [w584]
                        shift-right: [w586] -> w577
                        shift-left: w578 -> [w587]
                        i -> [w581]
                        n273 = Bundle By Name(cluster=T9 {"Test"={"Target Load"=0.0, "Target Disp"=0.0, "Rate"=0.0, "Speed"=0.0}, "Sensor"={"Name"=[], "Unit"=[], "Decimal Point"=[], "Ch Log"=[], "H Alarm"=[], "L Alarm"=[], "H Limit"=[], "L Limit"=[], "Filter"=[], "Gain"=[], "Calib Type"=[]}, "PID"={"SP"=-2.7823365e-08, "PV"=-3.023652e-13, "kP"=8.5432666e-24, "kI"=2.29252e-41, "kD"=1.570387e-38, "FF"=25.0, "Err Band"=0.0, "Max"=15, "Min"=-7, "Ts"=1886611780, "Out"=0, "Mode"=0}, "ADC"={"Active Ch"=[255, 255, 255, 0, 0, 0, 0, 0], "Filter Type"=2, "Post Filter"=[1, 1, 1, 1, 0, 200, 66, 184], "Gain"=[0, 0, 0, 0, 0, 122, 68, 0], "FS"=32, "IntOC"=0, "IntFC"=255, "SysOC"=255, "Cofficient"=[1.0, 1.0, 1.0, 1.0, 1.0, 1.0, 1.0, 1.0], "K"=[1.2450000047683716, 1.2450000047683716], "Max"=1048576}, "System"={"Out Type"=0, "Inverse"=0, "Monitor"=0, "Reserve"=0, "ACC Time"=0, "Pulse Rev"=0, "Stroke"=0, "Auto Off"=0, "Gear Ratio"=0.0, "Pitch"=0.0, "Max Speed"=0, "Jog Speed"=0, "Disp Coff"=0.0, "Max Load"=0}, "Index"=enum."Ch1", "Datalog"=enum."Empty"} ("Data"), "Index"=w581) -> (w580:T9)
                        n274 = call "UDP - Write CMD.vi"("V2"=TRUE, "CMD"=UDP_-_Command."Read Datalog Sensor", "error in"=w587, "Data"=w580, "UDP Info"=w584) -> ("error out"=w586:errorcluster)  [unwired: 6 out]
                        n275 = Wait (ms)(milliseconds to wait=u32 10) -> ()  [unwired: 1 out]
                      }
                    }
                  }
                }
              }
            }
          }
          frame "Close" {
            n276 = control-ref of="This VI"() -> (w590:refnum<vi>)
            n277 = invoke class="VI" method="FP.Close"(reference=w590, error in=w592) -> (error out=w593:errorcluster)  [unwired: 1 in, 2 out]
            n278 = call <vilib>:"Clear Errors.vi"("error in (no error)"=w593) -> ("error out"=w588:errorcluster)  [unwired: 5 in, 1 out]
          }
          frame "Exit" {
            n279 = control-ref of="This VI"() -> (w596:refnum<vi>)
            n280 = invoke class="VI" method="FP.Close"(reference=w596, error in=w597) -> (error out=w598:errorcluster)  [unwired: 1 in, 2 out]
          }
        }
      }
      frame Error {
        w607 = " - " ("string")
        n281 = call <vilib>:"Clear Errors.vi"("error in (no error)"=w611) -> ("error out"=w606:errorcluster)  [unwired: 5 in, 1 out]
        n282 = Unbundle By Name(w611) -> ("source"=w610:string)
        n283 = Format Into String(error in=w606, w603) -> (resulting string=w604:string, error out=w605:errorcluster)  [unwired: 2 in]
        n284 = Concatenate Strings("Machine" ("string"), w607, w604, w607, w610) -> (w609:string)
        n285 = call "General - Error Log eFGV.vi"("eFGV States"=eFGV_States."Write", "error in (no error)"=w605, "Error In"=w609) -> ("error out"=w612:errorcluster)  [unwired: 6 in, 2 out]
        n286 = Wait (ms)(milliseconds to wait=u32 100) -> ()  [unwired: 1 out]
      }
    }
    "Loop" <- w6
  }
  "error out" <- w4
  n287 = while {
    shift-right: [w624] -> _
    shift-left: "error in" -> [w626]
    shift-right: [w622] -> _
    shift-left: w1 -> [w625]
    shift-right: [w621] -> _
    shift-left: _ -> [w620]
    shift-left: w1 -> [w619]
    i -> [w618]
    stop <- w623 stop-if-true
    n288 = case shown="No Error" w626 {
      selector: w626 -> [w634 w767]
      tunnel: w625 -> [w627 _]
      tunnel: [w633 w766] -> w624
      tunnel: [w632 _] -> w623
      tunnel: [w631 Machine-state."Read"] -> w622
      tunnel: [w630 w763] -> w621
      tunnel: w620 -> [w629 w763]
      tunnel: w619 -> [_ w762]
      frame No Error {
        n289 = global read "Global - Data UDP.vi" "V1"() -> (w628:bool)
        n290 = case shown="\"Idle\"" w627 {
          tunnel: w634 -> [w637 w658 w718]
          tunnel: [w641 w657 w717] -> w633
          tunnel: [_ _ w715] -> w632
          tunnel: [Machine-state."Read" w659 Machine-state."Idle"] -> w631
          tunnel: [0 w655 0] -> w630
          tunnel: w629 -> [_ w656 _]
          tunnel: w628 -> [_ w652 w712]
          frame "Init", Default {
            n291 = for {
              N: 16 -> [_]
              shift-right: [w647] -> w638
              shift-left: w637 -> [w646]
              i -> [w644]
              n292 = Bundle By Name(cluster=T22 {"Row"=0, "Column"=4} ("Active Cell:Active Cell"), "Row"=w644) -> (w642:T22)
              n293 = property on="Table" class="MCListbox (strict)"(error in=w646, "ActiveCell"=w642, "CellBG"=u32 16777226) -> (error out=w647:errorcluster)  [unwired: 1 in, 1 out]
            }
            n294 = disable-structure shown="Disabled" {
              disable-tunnel: w638 -> [w649 w651]
              disable-tunnel: [w648 w651] -> w641
              frame Disabled {
                n295 = global read "Global - Rendezvous.vi" "rendezvous"() -> (w650:T11)
                n296 = call <vilib>:"Wait at Rendezvous.vi"("error in (no error)"=w649, "rendezvous"=w650) -> ("error out"=w648:errorcluster)  [unwired: 3 in, 2 out]
              }
              frame Enabled {
              }
            }
            n297 = Wait (ms)(milliseconds to wait=u32 100) -> ()  [unwired: 1 out]
          }
          frame "Idle" {
            n298 = Wait (ms)(milliseconds to wait=u32 250) -> ()  [unwired: 1 out]
            n299 = Increment(x=w656) -> (x+1=w655:i32)
            n300 = Greater Or Equal?(x=w655, y=4) -> (x >= y?=w653:bool)
            n301 = case shown="True" w652 {
              tunnel: [Machine-state."Read" ("f") w668] -> w659
              tunnel: w658 -> [w661 w667]
              tunnel: [w661 w666] -> w657
              tunnel: w653 -> [_ w664]
              frame False {
              }
              frame True {
                n302 = global read "Global - IP Address.vi" "IP"() -> (w672:string[])
                n303 = for {
                  tunnel: w672 -> [w673] mode=indexing
                  tunnel: [w677] -> w671 mode=indexing
                  shift-right: [w678] -> w666
                  shift-left: w667 -> [w675]
                  i -> [w676]
                  n304 = Empty String/Path?(string/path=w673) -> (empty?=w674:bool)
                  n305 = case shown="False" w674 {
                    tunnel: [w690 w711] -> w678
                    tunnel: [w689 TRUE ("Loop 16")] -> w677
                    tunnel: w676 -> [w687 _]
                    tunnel: w675 -> [w684 w711]
                    tunnel: w673 -> [w680 _]
                    frame False {
                      n306 = property on="Table" class="MCListbox (strict)"(error in=w684) -> (error out=w685:errorcluster, "ItemNames"=w683:string[][])  [unwired: 1 in, 1 out]
                      n307 = case shown="7" w687 {
                        tunnel: [w694 w695 w696 w697 w698 w699 w700 w701 w702 w703 w704 w705 w706 w707 w708 w709] -> w689
                        frame 0, Default {
                          n308 = global read "Global - Data UDP.vi" "Loop 1"() -> (w694:bool)
                        }
                        frame 1 {
                          n309 = global read "Global - Data UDP.vi" "Loop 2"() -> (w695:bool)
                        }
                        frame 2 {
                          n310 = global read "Global - Data UDP.vi" "Loop 3"() -> (w696:bool)
                        }
                        frame 3 {
                          n311 = global read "Global - Data UDP.vi" "Loop 4"() -> (w697:bool)
                        }
                        frame 4 {
                          n312 = global read "Global - Data UDP.vi" "Loop 5"() -> (w698:bool)
                        }
                        frame 5 {
                          n313 = global read "Global - Data UDP.vi" "Loop 6"() -> (w699:bool)
                        }
                        frame 6 {
                          n314 = global read "Global - Data UDP.vi" "Loop 7"() -> (w700:bool)
                        }
                        frame 7 {
                          n315 = global read "Global - Data UDP.vi" "Loop 8"() -> (w701:bool)
                        }
                        frame 8 {
                          n316 = global read "Global - Data UDP.vi" "Loop 9"() -> (w702:bool)
                        }
                        frame 9 {
                          n317 = global read "Global - Data UDP.vi" "Loop 10"() -> (w703:bool)
                        }
                        frame 10 {
                          n318 = global read "Global - Data UDP.vi" "Loop 11"() -> (w704:bool)
                        }
                        frame 11 {
                          n319 = global read "Global - Data UDP.vi" "Loop 12"() -> (w705:bool)
                        }
                        frame 12 {
                          n320 = global read "Global - Data UDP.vi" "Loop 13"() -> (w706:bool)
                        }
                        frame 13 {
                          n321 = global read "Global - Data UDP.vi" "Loop 14"() -> (w707:bool)
                        }
                        frame 14 {
                          n322 = global read "Global - Data UDP.vi" "Loop 15"() -> (w708:bool)
                        }
                        frame 15 {
                          n323 = global read "Global - Data UDP.vi" "Loop 16"() -> (w709:bool)
                        }
                      }
                      n324 = Index Array(array=w683, index (col)=0 ("disabled index (col)")) -> (element=w681:string[])  [unwired: 1 in]
                      n325 = Search 1D Array(1D array=w681, element=w680) -> (index of element=w679:i32)  [unwired: 1 in]
                      n326 = Bundle By Name(cluster=T22 {"Row"=0, "Column"=4} ("Active Cell:Active Cell"), "Row"=w679) -> (w686:T22)
                      n327 = Select(t=u32 6618880, s=w689, f=u32 16777226) -> (s? t:f=w691:u32)
                      n328 = property on="Table" class="MCListbox (strict)"(error in=w685, "ActiveCell"=w686, "CellBG"=w691) -> (error out=w690:errorcluster)  [unwired: 1 in, 1 out]
                    }
                    frame True {
                    }
                  }
                }
                n329 = And Array Elements(Boolean array=w671) -> (logical AND=w665:bool)
                n330 = Or(x=w664, y=w665) -> (x .or. y?=w663:bool)
                n331 = Select(t=Machine-state."Read", s=w663, f=Machine-state."Idle") -> (s? t:f=w668:T1)
              }
            }
          }
          frame "Read" {
            n332 = case shown="True" w712 {
              tunnel: w718 -> [w719 w725]
              tunnel: [w719 w724] -> w717
              frame False {
              }
              frame True {
                n333 = local read "Device Type"() -> (w720:string[])
                n334 = local read "Device IP"() -> (w721:string[])
                n335 = global read "Global - IP Address.vi" "IP"() -> (w722:string[])
                n336 = for {
                  tunnel: TRUE ("Bypass?") -> [w731]
                  tunnel: w722 -> [w726] mode=indexing
                  shift-right: [w732] -> w724
                  shift-left: w725 -> [w728]
                  tunnel: w721 -> [w730]
                  tunnel: w720 -> [w729]
                  i -> [w727]
                  n337 = case shown="Default" w726 {
                    selector: w726 -> [_ w734]
                    tunnel: [w733 w745] -> w732
                    tunnel: w731 -> [_ w744]
                    tunnel: w730 -> [_ w742]
                    tunnel: w729 -> [_ w741]
                    tunnel: w728 -> [w733 w736]
                    tunnel: w727 -> [_ w735]
                    frame "" {
                    }
                    frame Default {
                      n338 = Search 1D Array(1D array=w742, element=w734) -> (index of element=w740:i32)  [unwired: 1 in]
                      n339 = Index Array(array=w741, index=w740) -> (element=w739:string)
                      n340 = Equal?(x="Datalogger" ("y"), y=w739) -> (x = y?=w737:bool)
                      n341 = call "Communication - Send Command Read.vi"("Datalog?"=w737, "Bypass?"=w744, "error in (no error)"=w736, "Action"=UDP_-_Command."Read Ch Data", "Device IP Address"=w734) -> ("error out"=w745:errorcluster)  [unwired: 6 in]
                      n342 = case shown="0, Default" w735 {
                        frame 0, Default {
                          n343 = global write "Global - Data UDP.vi" "Loop 1"(FALSE ("Loop 1")) -> ()
                        }
                        frame 1 {
                          n344 = global write "Global - Data UDP.vi" "Loop 2"(FALSE ("Loop 2")) -> ()
                        }
                        frame 2 {
                          n345 = global write "Global - Data UDP.vi" "Loop 3"(FALSE ("Loop 3")) -> ()
                        }
                        frame 3 {
                          n346 = global write "Global - Data UDP.vi" "Loop 4"(FALSE ("Loop 4")) -> ()
                        }
                        frame 4 {
                          n347 = global write "Global - Data UDP.vi" "Loop 5"(FALSE ("Loop 5")) -> ()
                        }
                        frame 5 {
                          n348 = global write "Global - Data UDP.vi" "Loop 6"(FALSE ("Loop 6")) -> ()
                        }
                        frame 6 {
                          n349 = global write "Global - Data UDP.vi" "Loop 7"(FALSE ("Loop 7")) -> ()
                        }
                        frame 7 {
                          n350 = global write "Global - Data UDP.vi" "Loop 8"(FALSE ("Loop 8")) -> ()
                        }
                        frame 8 {
                          n351 = global write "Global - Data UDP.vi" "Loop 9"(FALSE ("Loop 9")) -> ()
                        }
                        frame 9 {
                          n352 = global write "Global - Data UDP.vi" "Loop 10"(FALSE ("Loop 10")) -> ()
                        }
                        frame 10 {
                          n353 = global write "Global - Data UDP.vi" "Loop 11"(FALSE ("Loop 11")) -> ()
                        }
                        frame 11 {
                          n354 = global write "Global - Data UDP.vi" "Loop 12"(FALSE ("Loop 12")) -> ()
                        }
                        frame 12 {
                          n355 = global write "Global - Data UDP.vi" "Loop 13"(FALSE ("Loop 13")) -> ()
                        }
                        frame 13 {
                          n356 = global write "Global - Data UDP.vi" "Loop 14"(FALSE ("Loop 14")) -> ()
                        }
                        frame 14 {
                          n357 = global write "Global - Data UDP.vi" "Loop 15"(FALSE ("Loop 15")) -> ()
                        }
                        frame 15 {
                          n358 = global write "Global - Data UDP.vi" "Loop 16"(FALSE ("Loop 16")) -> ()
                        }
                      }
                    }
                  }
                }
              }
            }
            n359 = call "General - Exit eFGV.vi"("eFGV States"=eFGV_States."Read") -> ("Exit Out"=w715:bool)  [unwired: 8 in, 2 out]
          }
        }
        "Enum 2" <- w627
      }
      frame Error {
        w772 = " - " ("string")
        n360 = call <vilib>:"Clear Errors.vi"("error in (no error)"=w767) -> ("error out"=w773:errorcluster)  [unwired: 5 in, 1 out]
        n361 = Unbundle By Name(w767) -> ("source"=w769:string)
        n362 = Format Into String(error in=w773, w762) -> (resulting string=w775:string, error out=w774:errorcluster)  [unwired: 2 in]
        n363 = Concatenate Strings("Machine2" ("string"), w772, w775, w772, w769) -> (w770:string)
        n364 = call "General - Error Log eFGV.vi"("eFGV States"=eFGV_States."Write", "error in (no error)"=w774, "Error In"=w770) -> ("error out"=w766:errorcluster)  [unwired: 6 in, 2 out]
        n365 = Wait (ms)(milliseconds to wait=u32 100) -> ()  [unwired: 1 out]
      }
    }
    "Numeric" <- w618
  }
